vi "Configure Power.vi"(0 "VISA resource name":refnum<visa-resource-name>, 1 "Power Reference (0 dBm)":dbl, 2 "Enable Power Reference (F:Disable)":bool, 5 "Power (-130 dBm)":dbl=-130.0, 7 "Power Offset (0 dB)":dbl, 9 "Attenuator Auto Mode (T:Enable)":bool=TRUE, 11 "error in (no error)":errorcluster, 12 "Enable Attenuator Bypass (F:Disable)":bool, 13 "Attenuation Level (115 dB)":dbl=115.0) -> (4 "VISA resource name out":refnum<visa-resource-name>, 15 "error out":errorcluster)   [LabVIEW 2018, in "Agilent PSG MXG Series.lvlib"]
doc: "Configures RF output power."
uses:
  Agilent PSG MXG Series.lvlib
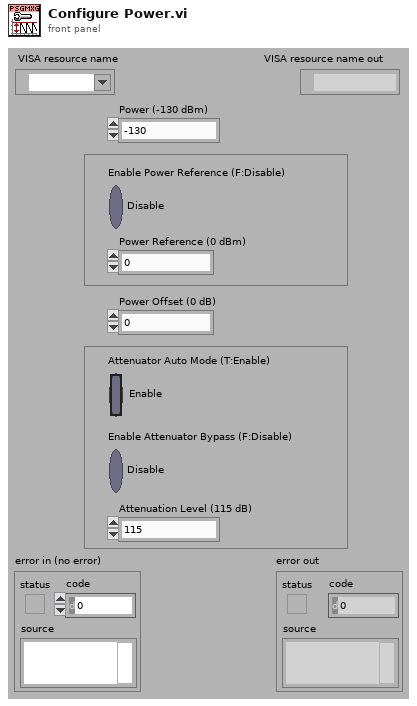
[diagram p1: front panel]
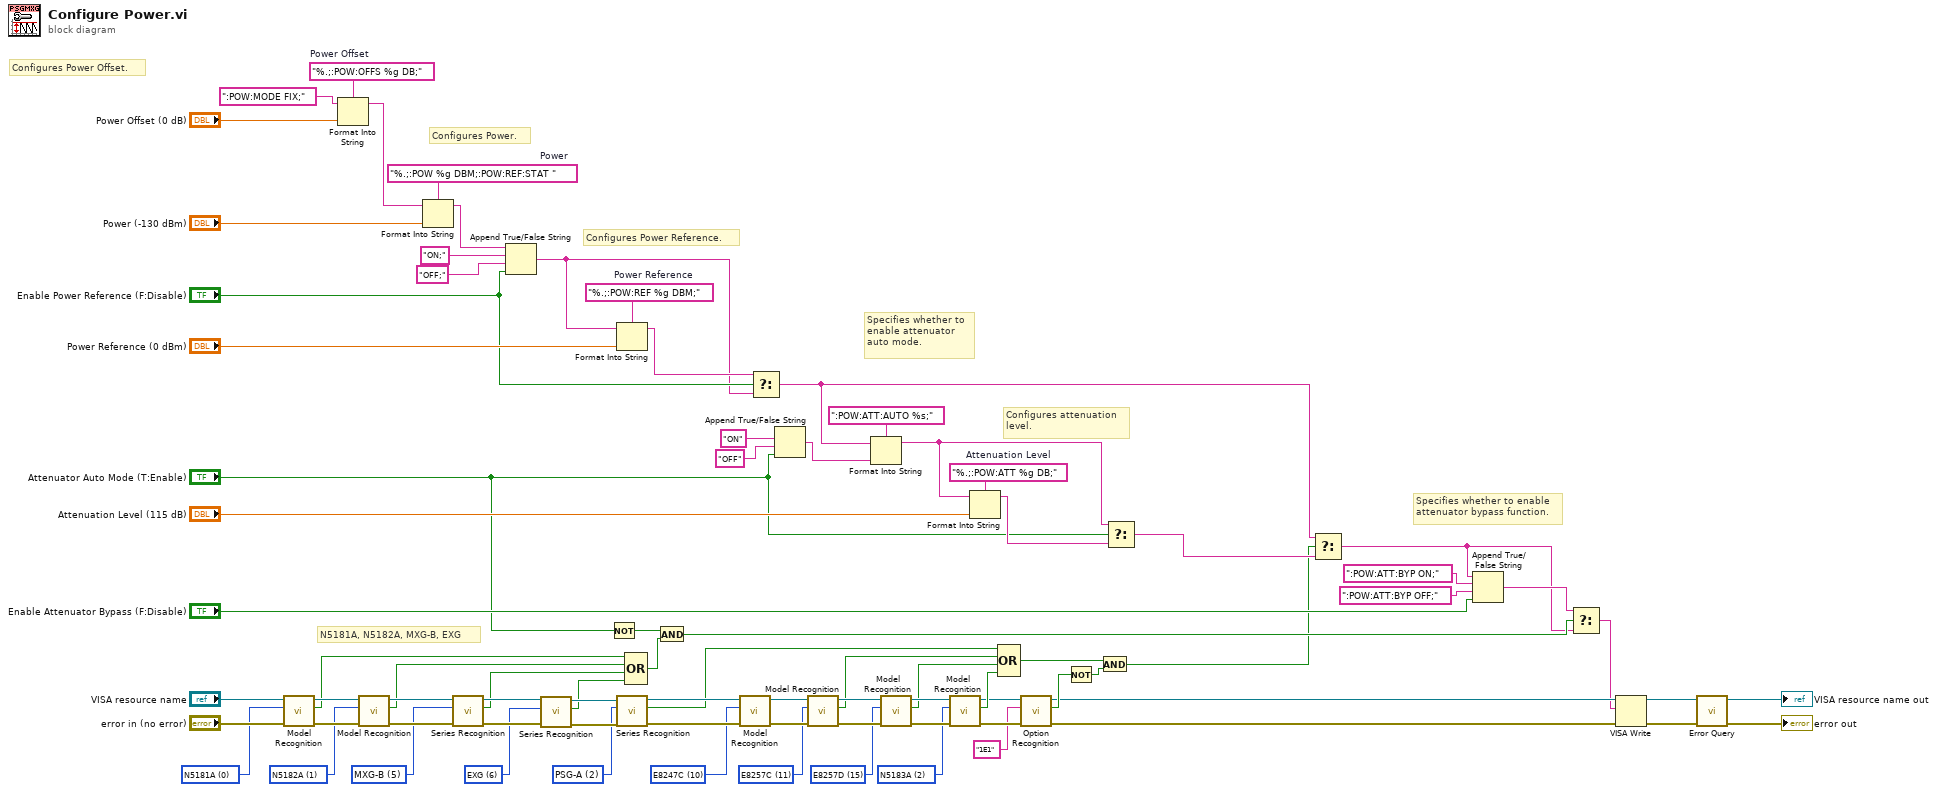
[diagram p0: block diagram]
diagram:
  w7 = u16 2 items=["N5181A"=0, "N5182A"=1, "N5183A"=2, "N5161A"=3, "N5162A"=4, "E8241A"=5, "E8244A"=6, "E8251A"=7, "E8254A"=8, "E8247C"=10, "E8257C"=11, "E8267C"=12, "E8257D"=15, "E8267D"=16, "N5171B"=17, "N5172B"=18, "N5181B"=19, "N5182B"=20] ("Model Type (0: N5181A)")
  w8 = u16 15 items=["N5181A"=0, "N5182A"=1, "N5183A"=2, "N5161A"=3, "N5162A"=4, "E8241A"=5, "E8244A"=6, "E8251A"=7, "E8254A"=8, "E8247C"=10, "E8257C"=11, "E8267C"=12, "E8257D"=15, "E8267D"=16, "N5171B"=17, "N5172B"=18, "N5181B"=19, "N5182B"=20] ("Model Type (0: N5181A)")
  w9 = u16 11 items=["N5181A"=0, "N5182A"=1, "N5183A"=2, "N5161A"=3, "N5162A"=4, "E8241A"=5, "E8244A"=6, "E8251A"=7, "E8254A"=8, "E8247C"=10, "E8257C"=11, "E8267C"=12, "E8257D"=15, "E8267D"=16, "N5171B"=17, "N5172B"=18, "N5181B"=19, "N5182B"=20] ("Model Type (0: N5181A)")
  w10 = u16 10 items=["N5181A"=0, "N5182A"=1, "N5183A"=2, "N5161A"=3, "N5162A"=4, "E8241A"=5, "E8244A"=6, "E8251A"=7, "E8254A"=8, "E8247C"=10, "E8257C"=11, "E8267C"=12, "E8257D"=15, "E8267D"=16, "N5171B"=17, "N5172B"=18, "N5181B"=19, "N5182B"=20] ("Model Type")
  w11 = u16 2 items=["MXG-A", "PSG", "PSG-A", "PSG-C", "PSG-D", "MXG-B", "EXG"] ("Series Type (0: MXG)")
  w18 = u16 6 items=["MXG-A", "PSG", "PSG-A", "PSG-C", "PSG-D", "MXG-B", "EXG"] ("Series Type (0: MXG)")
  w19 = u16 5 items=["MXG-A", "PSG", "PSG-A", "PSG-C", "PSG-D", "MXG-B", "EXG"] ("Series Type)")
  w26 = u16 1 items=["N5181A"=0, "N5182A"=1, "N5183A"=2, "N5161A"=3, "N5162A"=4, "E8241A"=5, "E8244A"=6, "E8251A"=7, "E8254A"=8, "E8247C"=10, "E8257C"=11, "E8267C"=12, "E8257D"=15, "E8267D"=16, "N5171B"=17, "N5172B"=18, "N5181B"=19, "N5182B"=20] ("Model Type (0: N5181A)")
  w27 = u16 0 items=["N5181A"=0, "N5182A"=1, "N5183A"=2, "N5161A"=3, "N5162A"=4, "E8241A"=5, "E8244A"=6, "E8251A"=7, "E8254A"=8, "E8247C"=10, "E8257C"=11, "E8267C"=12, "E8257D"=15, "E8267D"=16, "N5171B"=17, "N5172B"=18, "N5181B"=19, "N5182B"=20] ("Model Type")
  w61 = "%.;:POW:OFFS %g DB;"  # Power Offset
  w74 = "%.;:POW:ATT %g DB;"  # Attenuation Level
  w77 = "%.;:POW:REF %g DBM;"  # Power Reference
  w82 = "%.;:POW %g DBM;:POW:REF:STAT "  # Power
  # "N5181A, N5182A, MXG-B, EXG"
  # "Specifies whether to enable\nattenuator bypass function."
  # "Configures attenuation\nlevel."
  # "Specifies whether to\nenable attenuator\nauto mode."
  # "Configures Power Offset."
  # "Configures Power Reference."
  # "Configures Power."
  n1 = call "Model Recognition.vi"("error in (no error)"="error in (no error)", "Model Type (0: N5181A)"=w27, "VISA resource name"="VISA resource name") -> ("error out"=w52:errorcluster, "Is Model Correct"=w12:bool, "VISA resource name out"=w53:refnum<visa-resource-name>)  [unwired: 6 out]
  n2 = Format Into String(format string=w61, initial string=":POW:MODE FIX;" ("Power Mode"), "Power Offset (0 dB)") -> (resulting string=w28:string)  [unwired: 1 in, 1 out]
  n3 = call "Model Recognition.vi"("error in (no error)"=w52, "Model Type (0: N5181A)"=w26, "VISA resource name"=w53) -> ("error out"=w22:errorcluster, "Is Model Correct"=w13:bool, "VISA resource name out"=w25:refnum<visa-resource-name>)  [unwired: 6 out]
  n4 = Format Into String(format string=w82, initial string=w28, "Power (-130 dBm)") -> (resulting string=w80:string)  [unwired: 1 in, 1 out]
  n5 = call "Series Recognition.vi"("error in (no error)"=w22, "Series Type (0: MXG)"=w19, "VISA resource name"=w25) -> ("error out"=w21:errorcluster, "Is Series Correct"=w14:bool, "VISA resource name out"=w24:refnum<visa-resource-name>)  [unwired: 6 out]
  n6 = Append True/False String(1:"Enable Power Reference (F:Disable)", 2:"OFF;" ("false string"), 3:"ON;" ("true string"), 4:w80) -> (0:w63:string)
  n7 = call "Series Recognition.vi"("error in (no error)"=w21, "Series Type (0: MXG)"=w18, "VISA resource name"=w24) -> ("error out"=w20:errorcluster, "Is Series Correct"=w15:bool, "VISA resource name out"=w23:refnum<visa-resource-name>)  [unwired: 6 out]
  n8 = Not(x="Attenuator Auto Mode (T:Enable)") -> (.not. x?=w17:bool)
  n9 = Format Into String(format string=w77, initial string=w63, "Power Reference (0 dBm)") -> (resulting string=w64:string)  [unwired: 1 in, 1 out]
  n10 = call "Series Recognition.vi"("error in (no error)"=w20, "Series Type (0: MXG)"=w11, "VISA resource name"=w23) -> ("error out"=w50:errorcluster, "Is Series Correct"=w43:bool, "VISA resource name out"=w51:refnum<visa-resource-name>)  [unwired: 6 out]
  n11 = Compound Arithmetic op=OR(w12, w13, w14, w15) -> (w16:bool)
  n12 = And(x=w17, y=w16) -> (x .and. y?=w66:bool)
  n13 = call "Model Recognition.vi"("error in (no error)"=w50, "Model Type (0: N5181A)"=w10, "VISA resource name"=w51) -> ("error out"=w48:errorcluster, "VISA resource name out"=w49:refnum<visa-resource-name>)  [unwired: 7 out]
  n14 = Select(t=w64, s="Enable Power Reference (F:Disable)", f=w63) -> (s? t:f=w3:string)
  n15 = Append True/False String(1:"Attenuator Auto Mode (T:Enable)", 2:"OFF" ("false string"), 3:"ON" ("true string")) -> (0:w34:string)  [unwired: 1 out]
  n16 = call "Model Recognition.vi"("error in (no error)"=w48, "Model Type (0: N5181A)"=w9, "VISA resource name"=w49) -> ("error out"=w46:errorcluster, "Is Model Correct"=w42:bool, "VISA resource name out"=w47:refnum<visa-resource-name>)  [unwired: 6 out]
  n17 = Format Into String(format string=":POW:ATT:AUTO %s;", initial string=w3, w34) -> (resulting string=w33:string)  [unwired: 1 in, 1 out]
  n18 = call "Model Recognition.vi"("error in (no error)"=w46, "Model Type (0: N5181A)"=w8, "VISA resource name"=w47) -> ("error out"=w44:errorcluster, "Is Model Correct"=w41:bool, "VISA resource name out"=w45:refnum<visa-resource-name>)  [unwired: 6 out]
  n19 = call "Model Recognition.vi"("error in (no error)"=w44, "Model Type (0: N5181A)"=w7, "VISA resource name"=w45) -> ("error out"=w38:errorcluster, "Is Model Correct"=w40:bool, "VISA resource name out"=w39:refnum<visa-resource-name>)  [unwired: 6 out]
  n20 = Format Into String(format string=w74, initial string=w33, "Attenuation Level (115 dB)") -> (resulting string=w72:string)  [unwired: 1 in, 1 out]
  n21 = Compound Arithmetic op=OR(w43, w42, w41, w40) -> (w36:bool)
  n22 = call "Option Recognition.vi"("error in (no error)"=w38, "Option (\"\")"="1E1" ("Option (\"\")"), "VISA resource name"=w39) -> ("error out"=w4:errorcluster, "Is Option Installed"=w31:bool, "VISA resource name out"=w5:refnum<visa-resource-name>)  [unwired: 6 out]
  n23 = Not(x=w31) -> (.not. x?=w32:bool)
  n24 = And(x=w36, y=w32) -> (x .and. y?=w6:bool)
  n25 = Select(t=w33, s="Attenuator Auto Mode (T:Enable)", f=w72) -> (s? t:f=w30:string)
  n26 = Select(t=w3, s=w6, f=w30) -> (s? t:f=w2:string)
  n27 = Append True/False String(1:"Enable Attenuator Bypass (F:Disable)", 2:":POW:ATT:BYP OFF;" ("true string"), 3:":POW:ATT:BYP ON;" ("true string"), 4:w2) -> (0:w58:string)
  n28 = Select(t=w58, s=w66, f=w2) -> (s? t:f=w1:string)
  n29 = VISA Write(VISA resource name=w5, write buffer=w1, error in (no error)=w4) -> (VISA resource name out=w69:refnum<visa-resource-name>, error out=w68:errorcluster)  [unwired: 1 out]
  n30 = call "Error Query.vi"("error in (no error)"=w68, "VISA resource name"=w69) -> ("error out"=→"error out":errorcluster, "VISA resource name out"=→"VISA resource name out":refnum<visa-resource-name>)  [unwired: 8 out]
